vi "sest_test_I.vi"(8 "error in (no error)":errorcluster, 9 "table_length":i32, 10 "ISetOffset_mA":sgl, 11 "paramUnicorn_in":T1) -> (0 "error out":errorcluster, 3 "paramUnicorn_out":T1)   [LabVIEW 2017]
uses:
  Unicorn Labview Library/Control/unicorn_Param.ctl
  Unicorn Labview Library/Control/unicorn_conn.ctl
  Unicorn Labview Library/Control/unicorn_JSON.ctl
  Unicorn Labview Library/Control/unicorn_ParamInt.ctl
  Unicorn Labview Library/Control/unicorn_Telemetry.ctl
  Unicorn Labview Library/Control/unicorn_Table.ctl
  Unicorn Labview Library/Control/unicorn_ParamFloat.ctl
  Unicorn Labview Library/Unicorn Library.lvlib
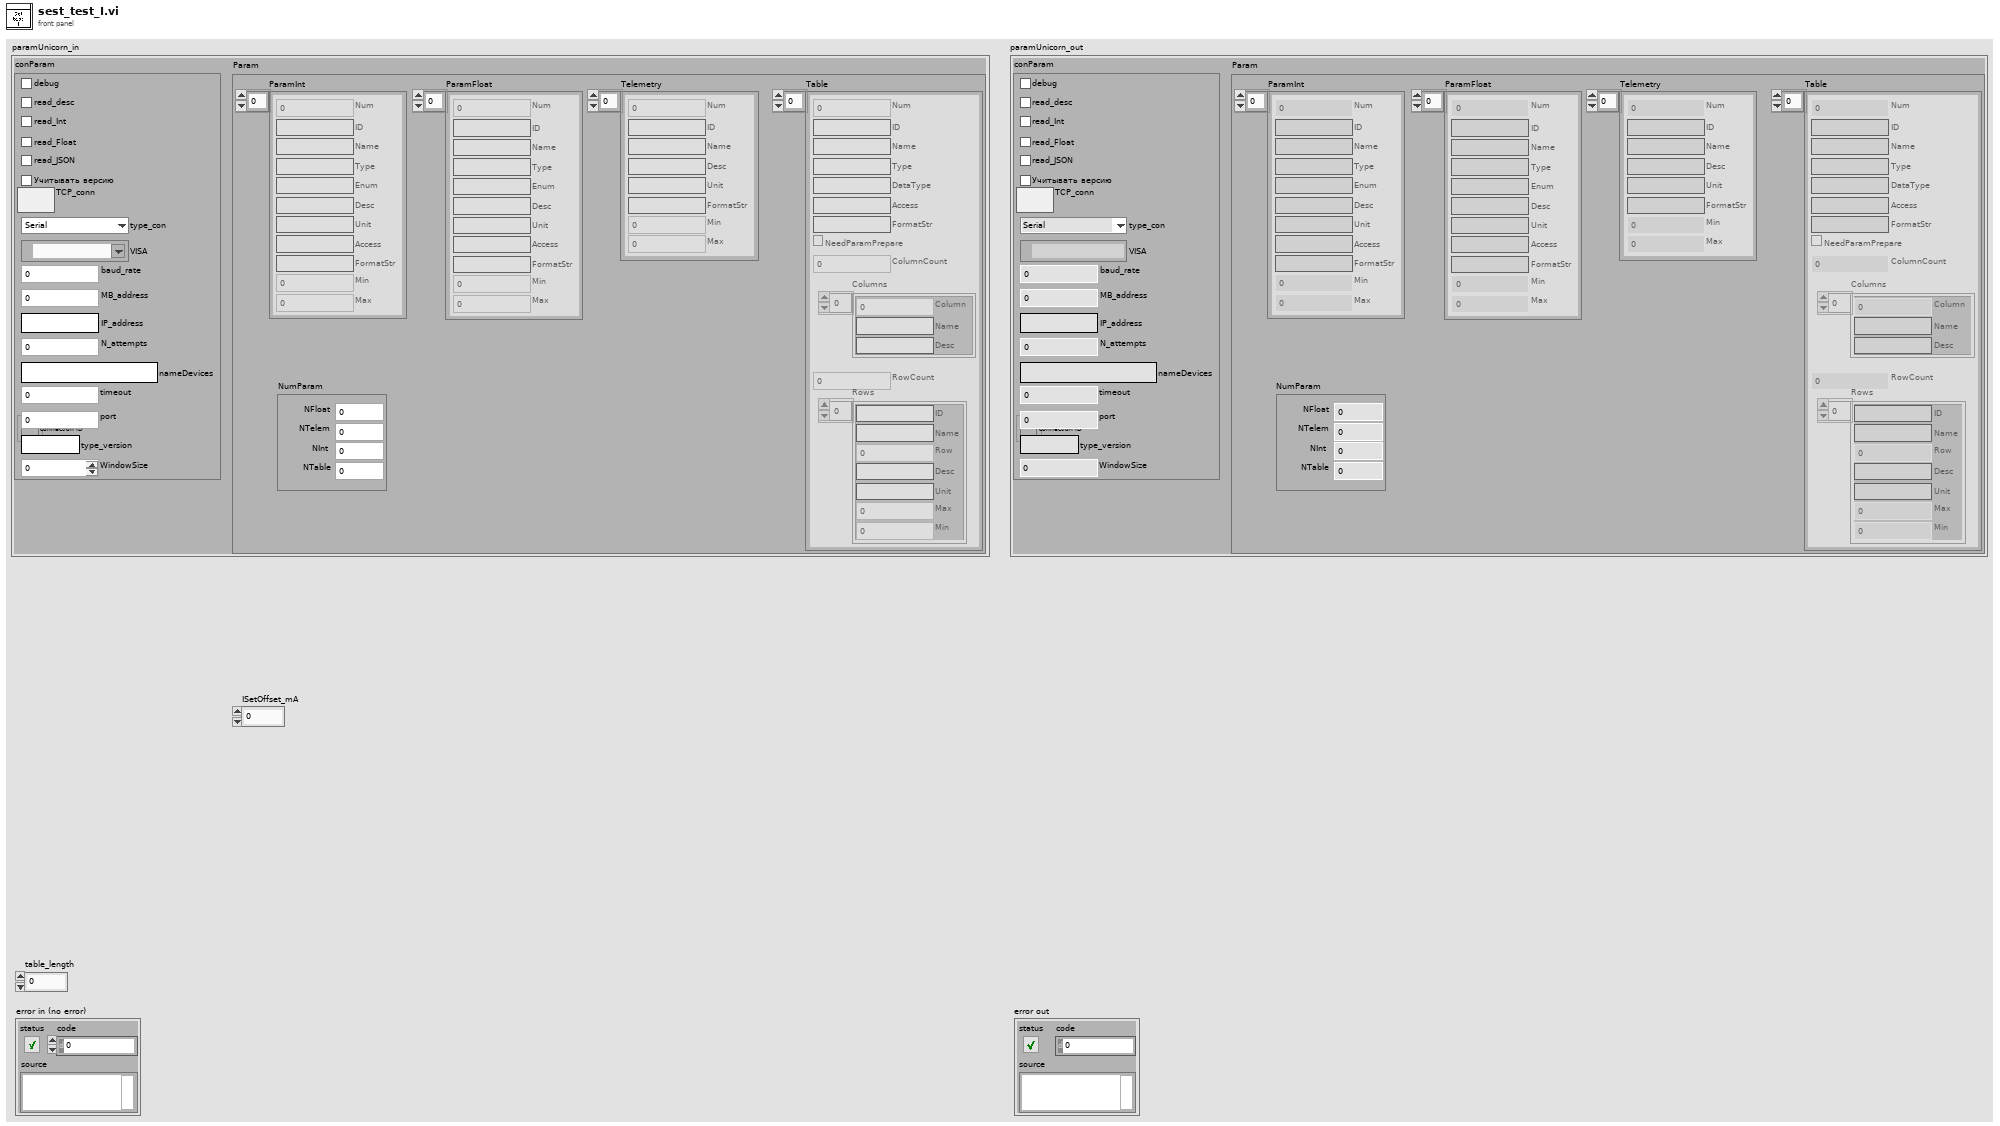
[diagram p1: front panel]
types:
  T1 = typedef "Unicorn Library.lvlib/unicorn_Param.ctl" = cluster{"conParam":T2, "Param":T3}
  T2 = typedef "Unicorn Library.lvlib/unicorn_conn.ctl" = cluster{"ReadIntParam":bool, "ReadDescrParam":bool, "ReadFloatParam":bool, "debug":bool, "ReadJSON":bool, "IP_address":string, "N_attempts":i32, "type_con":enum16{"Serial", "TCP"}, "MB_address":i32, "VISA":refnum<visa-resource-name>, "connection ID":refnum<k5>, "nameDevices":string, "timeout":i32, "port":u16, "type_version":string, "baud_rate":u32, "VersionControl":bool, "TCP_conn":bool, "WindowSize":i32}
  T3 = typedef "Unicorn Library.lvlib/unicorn_JSON.ctl" = cluster{"NumParam":cluster{"NTelem":i32, "NInt":i32, "NFloat":i32, "NTable":i32}, "ParamInt":T4, "Telemetry":T5, "Table":T6, "ParamFloat":T7}
  T4 = typedef "Unicorn Library.lvlib/unicorn_ParamInt.ctl" = cluster{"ID":string, "Num":i32, "Name":string, "Type":string, "Enum":string, "Desc":string, "Unit":string, "Access":string, "FormatStr":string, "Min":i32, "Max":i32}[]
  T5 = typedef "Unicorn Library.lvlib/unicorn_Telemetry.ctl" = cluster{"ID":string, "Num":i32, "Name":string, "Desc":string, "Unit":string, "FormatStr":string, "Min":i32, "Max":i32}[]
  T6 = typedef "Unicorn Library.lvlib/unicorn_Table.ctl" = cluster{"Num":i32, "Access":string, "ColumnCount":i32, "NeedParamPrepare":bool, "Columns":cluster{"Column":i32, "Desc":string, "Name":string}[], "DataType":string, "FormatStr":string, "ID":string, "Name":string, "RowCount":i32, "Rows":cluster{"Desc":string, "ID":string, "Max":i32, "Min":i32, "Name":string, "Row":i32, "Unit":string}[], "Type":string}[]
  T7 = typedef "Unicorn Library.lvlib/unicorn_ParamFloat.ctl" = cluster{"ID":string, "Num":i32, "Name":string, "Type":string, "Enum":string, "Desc":string, "Unit":string, "Access":string, "FormatStr":string, "Min":i32, "Max":i32}[]
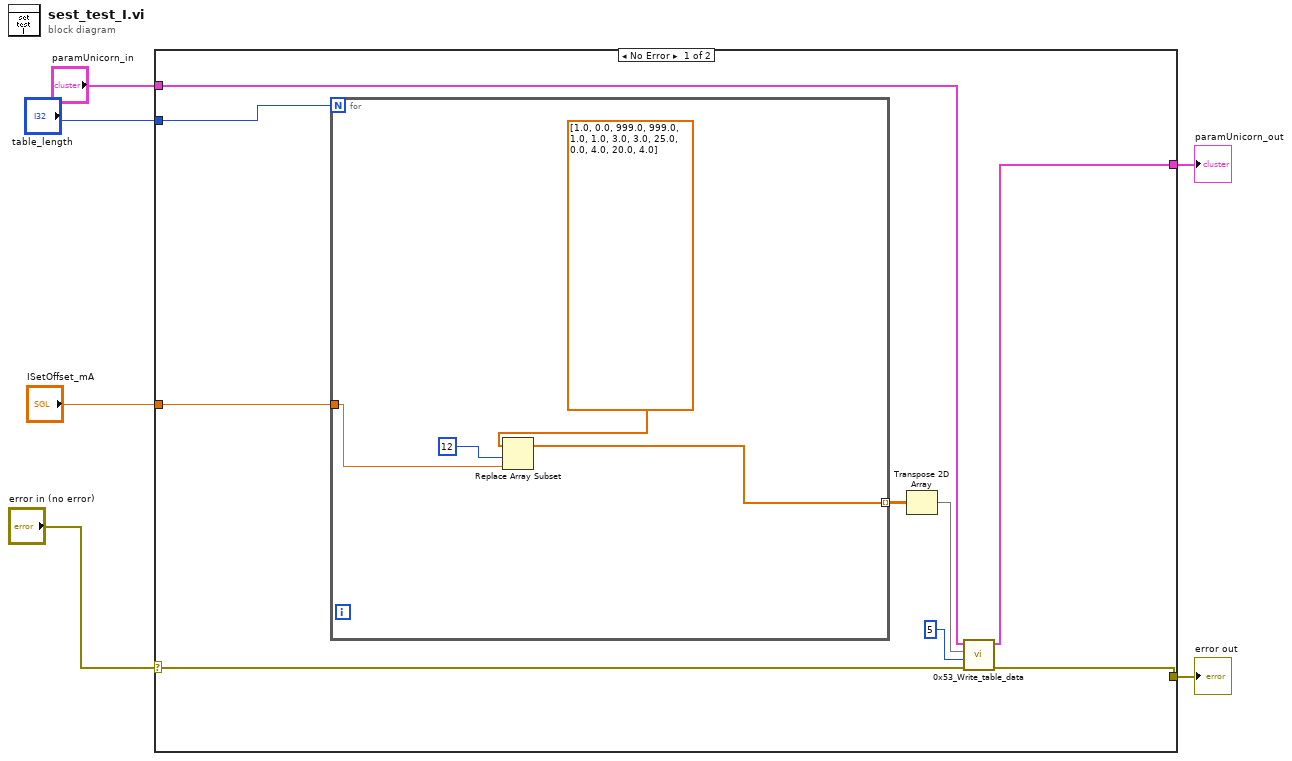
[diagram p0: block diagram]
diagram:
  n1 = case shown="No Error" "error in (no error)" {
    selector: "error in (no error)" -> [w9 w20]
    tunnel: "table_length" -> [w15 _]
    tunnel: "paramUnicorn_in" -> [w14 w21]
    tunnel: [w11 w21] -> w4
    tunnel: [w10 w20] -> w3
    tunnel: "ISetOffset_mA" -> [w7 _]
    frame No Error {
      n2 = for {
        N: w15 -> [_]
        tunnel: [w17] -> w8 mode=indexing
        tunnel: w7 -> [w16]
        n3 = Replace Array Subset "Replace Array Subset"(array=sgl[] [1.0, 0.0, 999.0, 999.0, 1.0, 1.0, 3.0, 3.0, 25.0, 0.0, 4.0, 20.0, 4.0] ("subarray"), new element=w16, index=12) -> (w17:sgl[])
      }
      n4 = Transpose 2D Array(2D array=w8) -> (transposed array=w13:sgl[][])
      n5 = call "0x53_Write_table_data.vi"("error in"=w9, "Номер табличного параметра 2"=5, "ArrayIn"=w13, "paramUnicorn"=w14) -> ("error out"=w10:errorcluster, "paramUnicorn 2"=w11:T1)  [unwired: 4 in, 2 out]
    }
    frame Error {
    }
  }
  "paramUnicorn_out" <- w4
  "error out" <- w3
